vi "FP_Move to Snap Location In WorkSpace.vi"(7 "WkSpace":T1, 8 "Error":errorcluster, 9 "Snap Location":T2, 11 "VI":refnum<vi>) -> (0 "Error Out":errorcluster, 3 "VI Out":refnum<vi>)   [LabVIEW 2025]
uses:
  TypeDefs_Utility/ENUM RB_Pos_Quadrant Position.ctl
  <vilib>/Utility/miscctls.llb/LVRectTypeDef.ctl
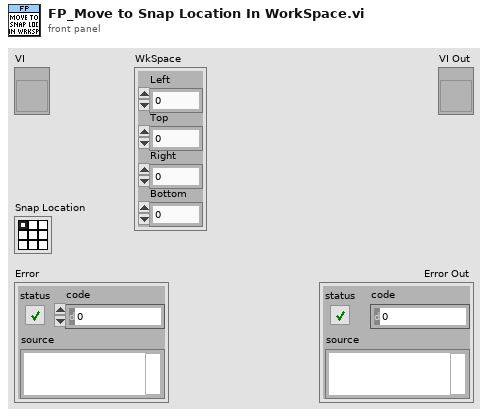
[diagram p1: front panel]
types:
  T1 = typedef "LVRectTypeDef.ctl" = cluster{"Left":i16, "Top":i16, "Right":i16, "Bottom":i16}
  T2 = typedef "ENUM RB_Pos_Quadrant Position.ctl" = enum32{"LFT-TOP", "MID-TOP", "RGT-TOP", "LFT-CTR", "MID-CTR", "RGT-CTR", "LFT-BOT", "MID-BOT", "RGT-BOT"}
  T3 = typedef "Cluster_Pos_Top Left position.ctl" = cluster{"Left":i16, "Top":i16}
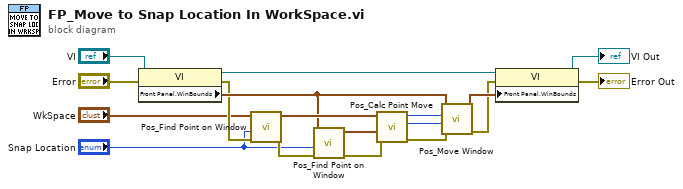
[diagram p0: block diagram]
diagram:
  n1 = property class="VI"(reference="VI", error in="Error") -> (reference out=w16:refnum<vi>, error out=w3:errorcluster, "Front Panel.WinBounds"=w6:T1)
  n2 = call "Pos_Find Point on Window.vi"("Error"=w3, "Position"="Snap Location", "Window"="WkSpace") -> ("Error Out"=w11:errorcluster, "Point Out"=w8:T3)  [unwired: 7 in]
  n3 = call "Pos_Find Point on Window.vi"("Error"=w11, "Position"="Snap Location", "Window"=w6) -> ("Error Out"=w12:errorcluster, "Point Out"=w7:T3)  [unwired: 7 in]
  n4 = call "Pos_Calc Point Move.vi"("Error"=w12, "Current Location"=w7, "Tartget Location"=w8) -> ("Error Out"=w13:errorcluster, "Down Out"=w10:i16, "Right Out"=w9:i16)  [unwired: 6 in]
  n5 = call "Pos_Move Window.vi"("Error"=w13, "Down"=w10, "Right"=w9, "Window"=w6) -> ("Error Out"=w4:errorcluster, "Window Out"=w5:T1)  [unwired: 6 in]
  n6 = property class="VI"(reference=w16, error in=w4, "Front Panel.WinBounds"=w5) -> (reference out=→"VI Out":refnum<vi>, error out=→"Error Out":errorcluster)
